vi "PlotDataTypes.vi"(1 "text":string, 2 "user-specified font":T4, 3 "alignment":T1={"horizontal"=enum."center", "vertical"=enum."center"}, 4 "desired font":T2(ring)=enum."System Font", 5 "rect":T3, 6 "point 2":cluster{"x":i16, "y":i16}, 7 "point":cluster{"x":i16, "y":i16}) -> (0 "Picture":picture)   [LabVIEW 2013]
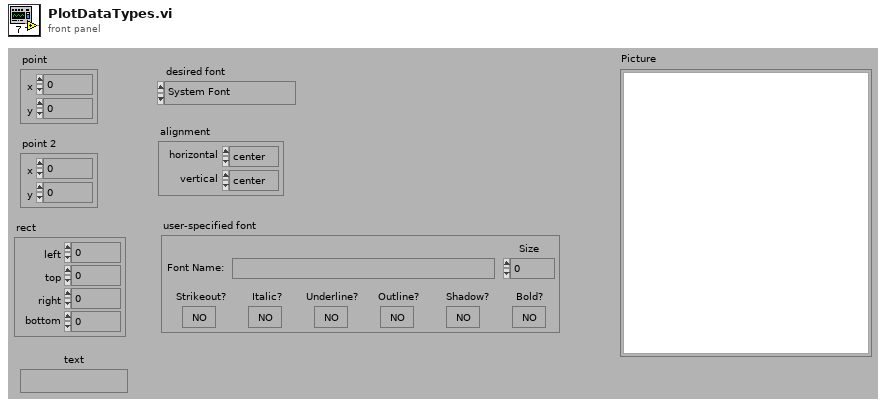
[diagram p1: front panel]
types:
  T1 = cluster{"horizontal":enum16{"left", "center", "right"}, "vertical":enum16{"top", "center", "bottom"}}
  T2 = enum16{"User-specified Font", "Application Font", "System Font", "Dialog Font"}
  T3 = cluster{"left":i16, "top":i16, "right":i16, "bottom":i16}
  T4 = cluster{"Font Name:":string, "Size":i16, "Strikeout?":bool, "Italic?":bool, "Underline?":bool, "Outline?":bool, "Shadow?":bool, "Bold?":bool}
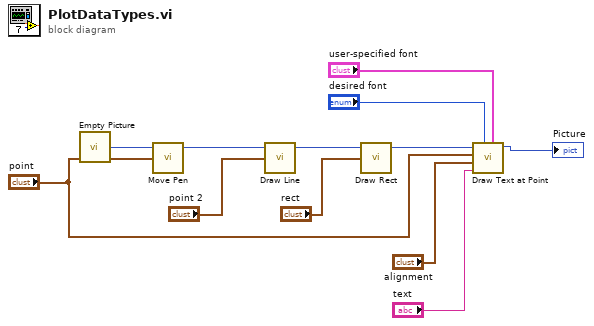
[diagram p0: block diagram]
diagram:
  n1 = call "Empty Picture"() -> ("empty picture"=w1:picture)
  n2 = call <vilib>:"Move Pen.vi"("new position"="point", "picture"=w1) -> ("new picture"=w12:picture)  [unwired: 1 in, 2 out]
  n3 = call <vilib>:"Draw Line.vi"("picture"=w12, "end point"="point 2") -> ("new picture"=w11:picture)  [unwired: 3 in, 4 out]
  n4 = call <vilib>:"Draw Rect.vi"("picture"=w11, "rect"="rect") -> ("new picture"=w9:picture)  [unwired: 3 in, 4 out]
  n5 = call <vilib>:"Draw Text at Point.vi"("[user-specified font]"="user-specified font", "desired font(Application)"="desired font", "text"="text", "alignment(left, top)"="alignment", "origin"="point", "picture"=w9) -> ("new picture"=→"Picture":picture)  [unwired: 3 in, 2 out]
